vi "LV9_5.vi"() -> ()   [LabVIEW 2011]
uses:
  <vilib>/imath/engines/lvmath2/RunTimeEngine/ErrorHandling/NIMS_Finalize Error.vi
  <vilib>/imath/engines/lvmath2/RunTimeEngine/NodeEndStatement/NIMS_NodeEndStatement_Output.vi
  <instcachedir>/0/NIMS_NodeEndStatement_Output_53EC0D466D134D7ABD903AC30B43404B.lvgen/NIMS_NodeEndStatement_Output_53EC0D466D134D7ABD903AC30B43404B_004.vi
  <instcachedir>/0/NIMS_NodeEndStatement_Output_53EC0D466D134D7ABD903AC30B43404B.lvgen/NIMS_NodeEndStatement_Output_53EC0D466D134D7ABD903AC30B43404B_005.vi
  <instcachedir>/0/NIMS_NodeEndStatement_Output_53EC0D466D134D7ABD903AC30B43404B.lvgen/NIMS_NodeEndStatement_Output_53EC0D466D134D7ABD903AC30B43404B_002.vi
  <vilib>/imath/engines/lvmath2/RunTimeEngine/ReplaceToken/NIMS_Replace - Check Linear.vi
  <instcachedir>/0/NIMS_Replace - Check Linear_276AD648BD064726893CCF9ED6E2A728.lvgen/NIMS_Replace - Check Linear_276AD648BD064726893CCF9ED6E2A728_007.vi
  <vilib>/imath/engines/lvmath2/RunTimeEngine/ReplaceToken/NIMS_Replace - Size Check _(_)=S.vi
  <instcachedir>/0/NIMS_Replace - Size Check _(_)=S_9ABE7AF2D26C43EAA05192D5C1E6C624.lvgen/NIMS_Replace - Size Check _(_)=S_9ABE7AF2D26C43EAA05192D5C1E6C624_005.vi
  <vilib>/imath/engines/lvmath2/RunTimeEngine/ReplaceToken/NIMS_Replace - V(S)=S.vi
  <instcachedir>/0/NIMS_Replace - V(S)=S_16B13A4565AB46F59881314645612498.lvgen/NIMS_Replace - V(S)=S_16B13A4565AB46F59881314645612498_002.vi
  <vilib>/imathl/engines/lvmath/Functions/Error Handling/Create Error.vi
  <vilib>/imath/engines/lvmath2/RunTimeEngine/RangeToken/NIMS_Range.vi
  <instcachedir>/0/NIMS_Range_0B7635FB69F84E19AA68E7FF959DF37C.lvgen/NIMS_Range_0B7635FB69F84E19AA68E7FF959DF37C_001.vi
  <vilib>/imath/engines/lvmath2/RunTimeEngine/ReplaceToken/NIMS_Replace - Check(_) Linear.vi
  <instcachedir>/0/NIMS_Replace - Check(_) Linear_271D1740B3B04FAC84D127F9D4901600.lvgen/NIMS_Replace - Check(_) Linear_271D1740B3B04FAC84D127F9D4901600_010.vi
  <instcachedir>/0/NIMS_Replace - Size Check _(_)=S_9ABE7AF2D26C43EAA05192D5C1E6C624.lvgen/NIMS_Replace - Size Check _(_)=S_9ABE7AF2D26C43EAA05192D5C1E6C624_007.vi
  <vilib>/imath/engines/lvmath2/RunTimeEngine/ReplaceToken/NIMS_Replace - V(V)=S.vi
  <instcachedir>/0/NIMS_Replace - V(V)=S_57753ECD8D164A28B5C1308A91DE1AEB.lvgen/NIMS_Replace - V(V)=S_57753ECD8D164A28B5C1308A91DE1AEB_002.vi
  <vilib>/imath/engines/lvmath2/RunTimeEngine/ErrorHandling/NIMS_Create Error From Enums.vi
  <vilib>/imath/engines/lvmath2/RunTimeEngine/BuiltInFunctions/randnormal/NIMS_randnormal(Str,I32).vi
  <vilib>/imath/engines/lvmath2/RunTimeEngine/BuiltInFunctions/randnormal/NIMS_randnormal(1,I32).vi
  <vilib>/imath/engines/lvmath2/RunTimeEngine/ArithmeticOperatorToken/NIMS_ArithmeticOperator_plus.vi
  <instcachedir>/0/NIMS_ArithmeticOperator_plus_1E95F7DAB906458CBECCADBE8E6FD739.lvgen/NIMS_ArithmeticOperator_plus_1E95F7DAB906458CBECCADBE8E6FD739_010.vi
  <vilib>/imath/engines/lvmath2/RunTimeEngine/RangeToken/NIMS_Range_R2.vi
  <instcachedir>/0/NIMS_Replace - Check Linear_276AD648BD064726893CCF9ED6E2A728.lvgen/NIMS_Replace - Check Linear_276AD648BD064726893CCF9ED6E2A728_008.vi
  <instcachedir>/0/NIMS_Replace - Size Check _(_)=S_9ABE7AF2D26C43EAA05192D5C1E6C624.lvgen/NIMS_Replace - Size Check _(_)=S_9ABE7AF2D26C43EAA05192D5C1E6C624_008.vi
  <vilib>/imath/engines/lvmath2/RunTimeEngine/ReplaceToken/NIMS_Replace - V(R2)=S.vi
  <instcachedir>/0/NIMS_Replace - V(R2)=S_820D79DEC52B4430A25BB746A47D1A64.lvgen/NIMS_Replace - V(R2)=S_820D79DEC52B4430A25BB746A47D1A64_002.vi
  <vilib>/imath/engines/lvmath2/RunTimeEngine/BuiltInFunctions/fft/NIMS_fft(GV).vi
  <instcachedir>/0/NIMS_fft(GV)_4C6467FC22F84E4BA42517A07EF978B0.lvgen/NIMS_fft(GV)_4C6467FC22F84E4BA42517A07EF978B0_000.vi
  <vilib>/imath/engines/lvmath2/RunTimeEngine/BuiltInFunctions/conjugate/NIMS_conjugate(Complex).vi
  <instcachedir>/0/NIMS_conjugate(Complex)_151E186CA54B4853A0120BB0A667D86E.lvgen/NIMS_conjugate(Complex)_151E186CA54B4853A0120BB0A667D86E_001.vi
  <vilib>/imath/engines/lvmath2/RunTimeEngine/ArithmeticOperatorToken/NIMS_ArithmeticOperator_times.vi
  <instcachedir>/0/NIMS_ArithmeticOperator_times_3FA9DDB491BD45F6905798C0465C9825.lvgen/NIMS_ArithmeticOperator_times_3FA9DDB491BD45F6905798C0465C9825_003.vi
  <vilib>/imath/engines/lvmath2/RunTimeEngine/BuiltInFunctions/ifft2d/NIMS_ifft2d.vi
  <vilib>/imath/engines/lvmath2/RunTimeEngine/ErrorHandling/NIMS_Error From Error Code.vi
  <vilib>/imath/engines/lvmath2/RunTimeEngine/VariableToken/Read/NIMS_Get Elements - SorM(_) - Check(_).vi
  <instcachedir>/0/NIMS_Get Elements - SorM(_) - Check(_)_561A7B7910804DA3BBA41B7F4E44AAB4.lvgen/NIMS_Get Elements - SorM(_) - Check(_)_561A7B7910804DA3BBA41B7F4E44AAB4_008.vi
  <instcachedir>/0/NIMS_Range_0B7635FB69F84E19AA68E7FF959DF37C.lvgen/NIMS_Range_0B7635FB69F84E19AA68E7FF959DF37C_000.vi
panel:
  in  "stop":bool
  in  "Noise level":dbl(slide) step=0.001 scale=0.0..1.5
  out "Signals":cluster{"T":dbl[], "X":dbl[]}[](graph)
  in  "Delay":dbl(slide) step=0.001 scale=0.1..0.4
  out "Cross-correlation":cluster{"TA":dbl[], "A":dbl[]}(graph)
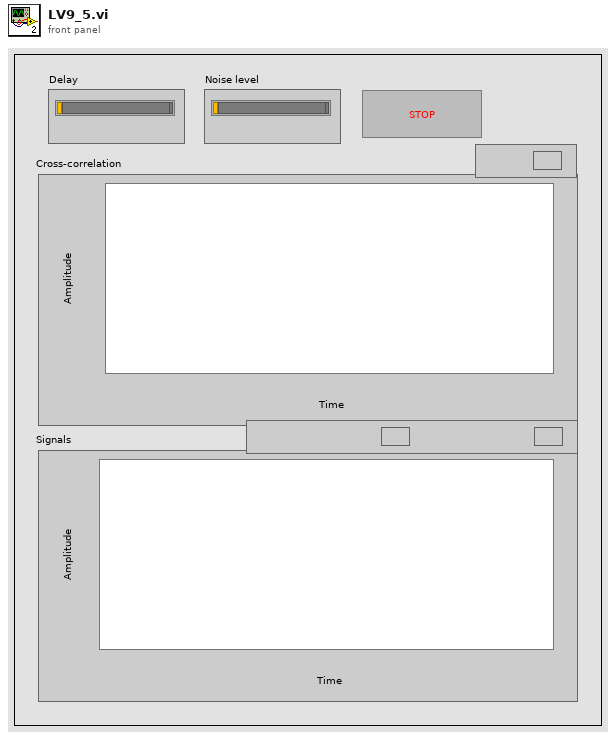
[diagram p1: front panel]
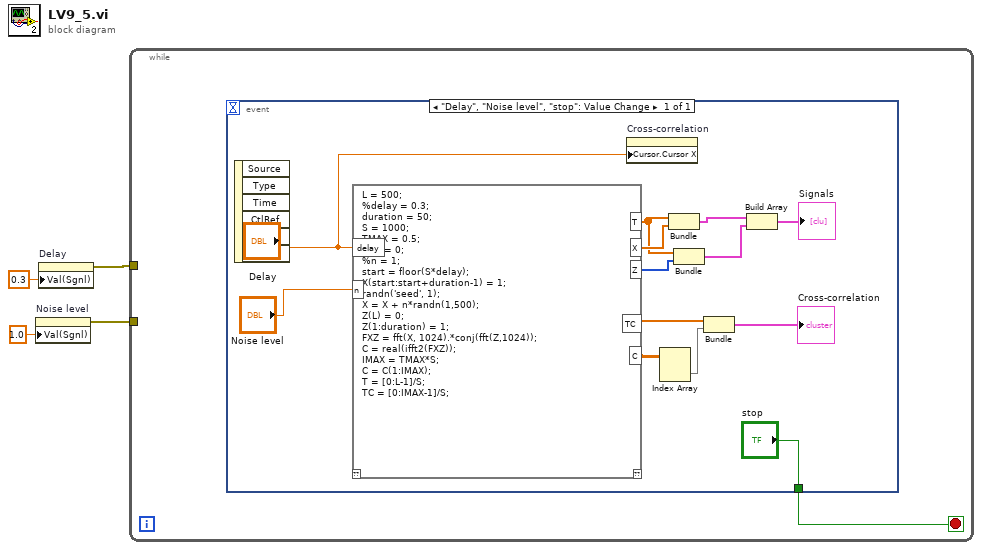
[diagram p0: block diagram]
diagram:
  n1 = property on="Noise level" class="Slide (strict)"("Val(Sgnl)"=1.0 ("Value (Signaling)")) -> (error out=w3:errorcluster)  [unwired: 2 in, 1 out]
  n2 = property on="Delay" class="Slide (strict)"("Val(Sgnl)"=0.3 ("Value (Signaling)")) -> (error out=w4:errorcluster)  [unwired: 2 in, 1 out]
  n3 = while {
    tunnel: w4 -> [_]
    tunnel: w3 -> [_]
    stop <- w5 stop-if-true
    n4 = event shown="[0] \"Delay\", \"Noise level\", \"stop\": Value Change" {
      selector: _ -> [_]
      dyn-events: _ -> [_]
      timeout: _ -> [_]
      tunnel: ["stop"] -> w5
      event "Delay", "Noise level", "stop": Value Change {
        n5 = event-data() -> ()  [unwired: 1 in, 6 out]
        n6 = mathscript code="L = 500;\n%delay = 0.3;\nduration = 50;\nS = 1000;\nTMAX = 0.5;\nX(L) = 0;\n%n = 1;\nstart = floor(S*delay);\nX(start:start+duration-1) = 1;\nrandn('seed', 1);\nX = X + n*randn(1,500);\nZ(L) = 0;\nZ(1:duration) = 1;\nFXZ = fft(X, 1024).*conj(fft(Z,1024));\nC = real(ifft2(FXZ));\nIMAX = TMAX*S;\nC = C(1:IMAX);\nT = [0:L-1]/S;\nTC = [0:IMAX-1]/S;"("delay"="Delay", "n"="Noise level") -> ("C"=w16:dbl[][], "TC"=w17:dbl[], "T"=w11:dbl[], "X"=w18:dbl[], "Z"=w10:i32[])  [unwired: 1 in, 1 out]
        n7 = property on="Cross-correlation" class="XYGraph (strict)"("Cursor.Cursor X"="Delay") -> ()  [unwired: 2 in, 2 out]
        n8 = Index Array(array=w16) -> (element=w15:dbl[])  [unwired: 2 in]
        n9 = Bundle("T"=w11, "X"=w18) -> (w9:cluster{"T":dbl[], "X":dbl[]})  [unwired: 1 in]
        n10 = Bundle("T"=w11, "Z"=w10) -> (w8:cluster{"T":dbl[], "Z":i32[]})  [unwired: 1 in]
        n11 = Bundle("TC"=w17, "C"=w15) -> (→"Cross-correlation":cluster{"TC":dbl[], "C":dbl[]})  [unwired: 1 in]
        n12 = Build Array(w9, w8) -> (→"Signals":cluster{"T":dbl[], "X":dbl[]}[])
      }
    }
  }
